vi "axex_test.vi"() -> ()   [LabVIEW 2020, in "AX Excel.lvlib"]
doc: "AX Excel demo VI."
uses:
  AX Excel.lvlib
  axex_cell_xy.ctl
  axex_write_cell.vi
  axex_read_cell.vi
panel:
  out "cell string out":string
  out "error out 2":errorcluster
  out "Numeric":i32
  in  "stop":bool
  in  "open active workbook (False)":bool
  in  "save path (no path)":path
  in  "window state":T1(ring)=enum."Don't change"
  out "error out":errorcluster
  in  "excel file path (full)":path
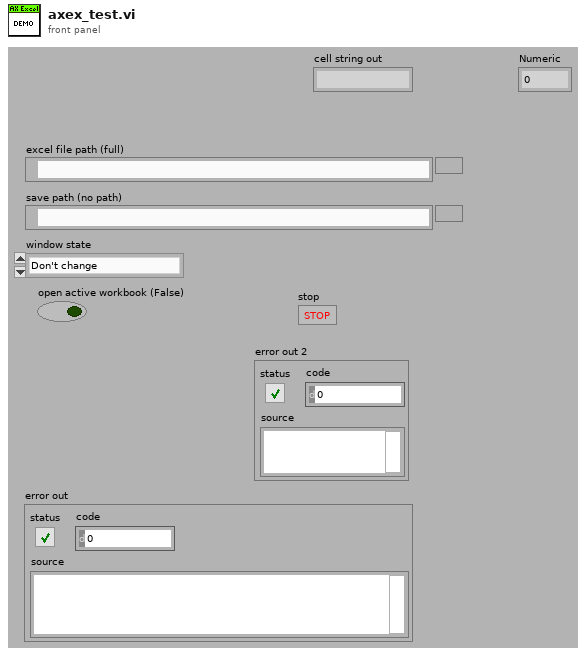
[diagram p1: front panel]
types:
  T1 = enum16{"Minimized", "Maximized", "Normal", "Don't change"}
  T2 = typedef "AX Excel.lvlib/axex_instance.ctl" = cluster{"file path":path, "current sheet name":string, "sheet ref":refnum<k7>, "wbook ref":refnum<k7>}
  T3 = typedef "AX Excel.lvlib/axex_cell_xy.ctl" = cluster{"column":i32, "row":i32, "cell name":string}
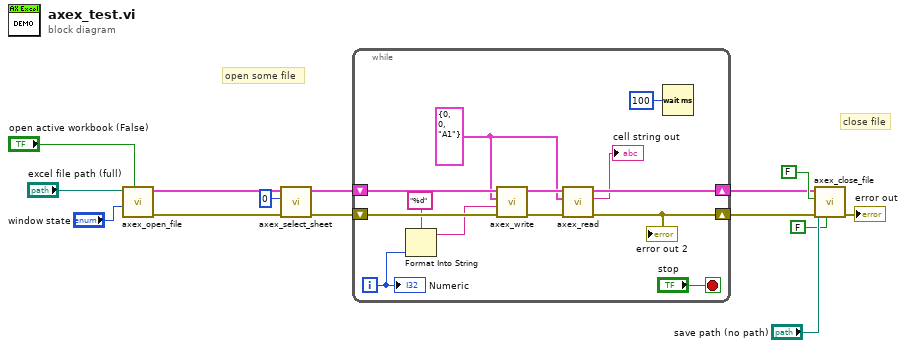
[diagram p0: block diagram]
diagram:
  # "close file"
  # "open some file"
  n1 = call "axex_open_file.vi"("open active workbook (False)"="open active workbook (False)", "window state (unchanged)"="window state", "excel file path (full)"="excel file path (full)") -> ("error out"=w5:errorcluster, "AX Excel instance out"=w2:T2)  [unwired: 7 in]
  n2 = call "axex_select_sheet.vi"("error in"=w5, "sheet id"=0, "AX Excel instance in"=w2) -> ("error out"=w4:errorcluster, "AX Excel instance out"=w3:T2)  [unwired: 5 in, 2 out]
  n3 = while {
    shift-right: [w18] -> w7
    shift-left: w4 -> [w24]
    shift-right: [w17] -> w6
    shift-left: w3 -> [w25]
    i -> [w23]
    stop <- "stop" stop-if-true
    w16 = T3 {"column"=0, "row"=0, "cell name"="A1"} ("cell")
    n4 = Format Into String(format string="%d", w23) -> (resulting string=w21:string)  [unwired: 2 in, 1 out]
    n5 = call-poly "axex_write.vi"("error in"=w24, "string"=w21, "cell"=w16, "AX Excel instance in"=w25) -> ("error out"=w20:errorcluster, "AX Excel instance out"=w19:T2)  [unwired: 6 in]
    n6 = call-poly "axex_read.vi"("error in"=w20, "cell"=w16, "AX Excel instance in"=w19) -> ("error out"=w18:errorcluster, "cell string out"=→"cell string out":string, "AX Excel instance out"=w17:T2)  [unwired: 6 in]
    "error out 2" <- w18
    n7 = Wait (ms)(milliseconds to wait=u32 100) -> ()  [unwired: 1 out]
    "Numeric" <- w23
  }
  n8 = call "axex_close_file.vi"("file overwrite prompt (True)"=FALSE, "error in"=w7, "save path (no path)"="save path (no path)", "save changes (True)"=FALSE, "AX Excel instance in"=w6) -> ("error out"=→"error out":errorcluster)  [unwired: 6 in]
